vi "choose firs acquisition state.vi"(8 "error in (no error)":errorcluster, 11 "Channel in":refnum<class "Channel.lvclass">) -> (0 "error out":errorcluster, 2 "next status":string, 3 "Channel out":refnum<class "Channel.lvclass">)   [LabVIEW 2018, in "Channel.lvclass"]
uses:
  Channel.lvclass
  Channel.lvclass/Channel.ctl
  Header content/Header content.lvclass/Header content.ctl
  Server/Server.lvclass/Server.ctl
  Server/Server.lvclass
  RxTx/CCS_RxTx.lvclass
  Header content/Header content.lvclass
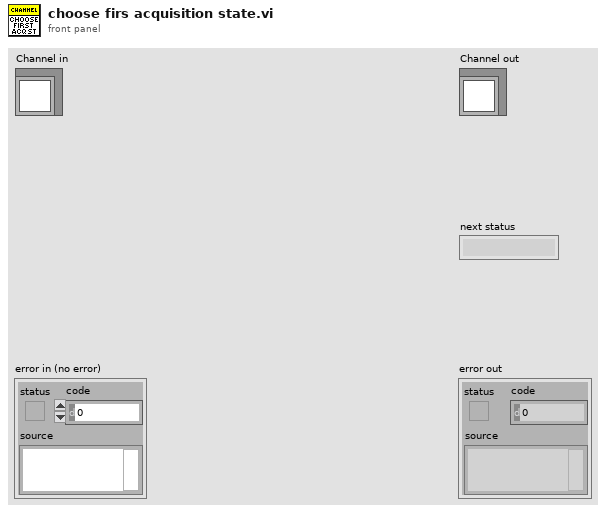
[diagram p1: front panel]
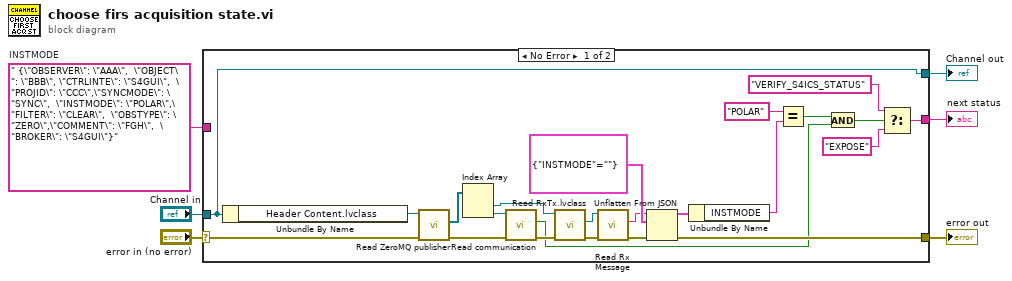
[diagram p0: block diagram]
diagram:
  w2 = " {\"OBSERVER\": \"AAA\",  \"OBJECT\": \"BBB\", \"CTRLINTE\": \"S4GUI\",  \"PROJID\": \"CCC\",\"SYNCMODE\": \"SYNC\",  \"INSTMODE\": \"POLAR\",\"FILTER\": \"CLEAR\",  \"OBSTYPE\": \"ZERO\",\"COMMENT\": \"FGH\",  \"BROKER\": \"S4GUI\"}"  # INSTMODE
  n1 = case shown="No Error" "error in (no error)" {
    selector: "error in (no error)" -> [w24 w31]
    tunnel: [w20 w31] -> w5
    tunnel: [w26 w30] -> w3
    tunnel: "Channel in" -> [w26 w30]
    tunnel: w2 -> [_ _]
    tunnel: [w8 _] -> w1
    frame No Error {
      n2 = Unbundle By Name(w26) -> ("Header Content.lvclass"=w25:refnum<class "Header content.lvclass">)
      n3 = call "Read ZeroMQ publisher.vi"("error in (no error)"=w24, "Header content in"=w25) -> ("error out"=w13:errorcluster, "ZeroMQ publisher"=w29:refnum<class "Server.lvclass">[])  [unwired: 7 in, 1 out]
      n4 = Index Array(array=w29) -> (element #1=w16:refnum<class "Server.lvclass">, element #2=w15:refnum<class "Server.lvclass">)  [unwired: 2 in]
      n5 = call "Read communication.vi"("error in (no error)"=w13, "Server in"=w15) -> ("error out"=w14:errorcluster, "communication"=w7:bool)  [unwired: 7 in, 1 out]
      n6 = call "Read RxTx.lvclass.vi"("error in (no error)"=w14, "Server in"=w16) -> ("error out"=w27:errorcluster, "RxTx.lvclass"=w28:refnum<class "CCS_RxTx.lvclass">)  [unwired: 7 in, 1 out]
      n7 = call "Read Rx Message.vi"("error in (no error)"=w27, "RxTx in"=w28) -> ("error out"=w23:errorcluster, "Rx Message"=w9:string)  [unwired: 7 in, 1 out]
      n8 = Unflatten From JSON(JSON string=w9, type and defaults=cluster{"INSTMODE":string} {"INSTMODE"=""}, error in (no error)=w23) -> (value=w22:cluster{"INSTMODE":string}, error out=w20:errorcluster)  [unwired: 4 in]
      n9 = Unbundle By Name(w22) -> ("INSTMODE"=w19:string)
      n10 = Equal?(x="POLAR", y=w19) -> (x = y?=w17:bool)
      n11 = And(x=w17, y=w7) -> (x .and. y?=w12:bool)
      n12 = Select(t="VERIFY_S4ICS_STATUS" ("x"), s=w12, f="EXPOSE" ("x")) -> (s? t:f=w8:string)
    }
    frame Error {
    }
  }
  "error out" <- w5
  "Channel out" <- w3
  "next status" <- w1
